vi "Get Hwnd.vi"(8 "error in (no error)":errorcluster, 10 "Doc Name":string) -> (0 "error out":errorcluster, 2 "hwnd":u32)   [LabVIEW 2016, in "Document.lvclass"]
uses:
  Document.lvclass
  user32.dll
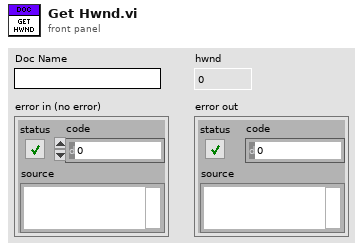
[diagram p1: front panel]
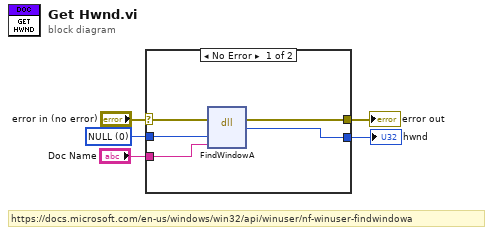
[diagram p0: block diagram]
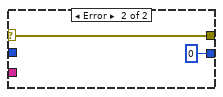
[diagram p2: hidden frame]
diagram:
  w1 = 0 items=["NULL"]
  # "https://docs.microsoft.com/en-us/windows/win32/api/winuser/nf-winuser-findwindowa"
  n1 = case shown="No Error" "error in (no error)" {
    selector: "error in (no error)" -> [w10 w12]
    tunnel: "Doc Name" -> [w9 _]
    tunnel: [w8 u32 0 ("hwnd")] -> w3
    tunnel: [w7 w12] -> w2
    tunnel: w1 -> [w6 _]
    frame No Error {
      n2 = dll-call lib="user32.dll" fn="FindWindowA"(error in=w10, "lpzsClassName"=w6, "lpzsWindowName"=w9) -> (error out=w7:errorcluster, "hwnd"=w8:u32)  [unwired: 4 in, 1 out]
    }
    frame Error {
    }
  }
  "hwnd" <- w3
  "error out" <- w2
